vi "Write Lookup Tables.vi"(8 "error in (no error)":errorcluster, 10 "Lookup Tables":T1[](array[typedef]), 11 "Plugin_UI in":refnum<class "Plugin_UI.lvclass">) -> (0 "error out":errorcluster, 3 "Plugin_UI out":refnum<class "Plugin_UI.lvclass">)   [LabVIEW 2020, in "Plugin.lvlib" / "Plugin_UI.lvclass"]
doc: "Write lookup table"
uses:
  Plugin_UI.lvclass
  builds/Libraries/LabSys Framework.lvlibp/Configuration Storage/Test Configuration/Table Information.ctl
  Plugin_UI.lvclass/Plugin_UI.ctl
  builds/Libraries/LabSys Framework.lvlibp/Configuration Storage/Test Configuration/Test Configuration.lvclass
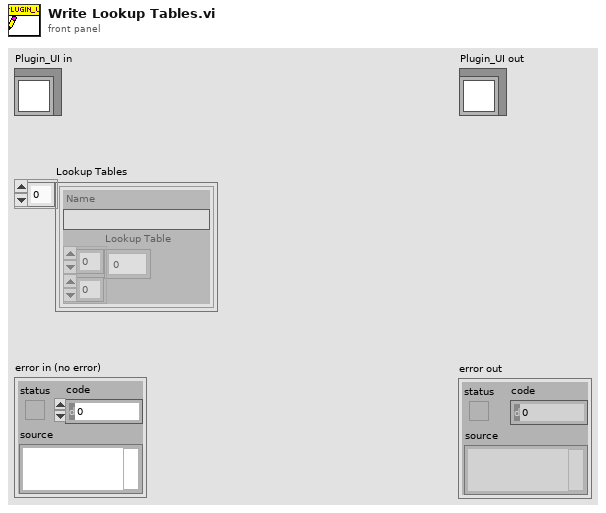
[diagram p1: front panel]
types:
  T1 = typedef "LabSys Framework.lvlibp/Configuration Storage.lvlib/Test Configuration.lvclass/Table Information.ctl" = cluster{"Name":string, "Lookup Table":dbl[][]}
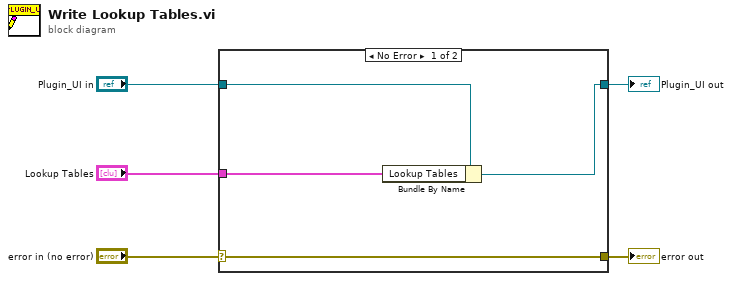
[diagram p0: block diagram]
diagram:
  n1 = case shown="No Error" "error in (no error)" {
    selector: "error in (no error)" -> [w9 w10]
    tunnel: [w9 w10] -> w4
    tunnel: [w7 w11] -> w2
    tunnel: "Plugin_UI in" -> [w8 w11]
    tunnel: "Lookup Tables" -> [w6 _]
    frame No Error {
      n2 = Bundle By Name(cluster=w8, "Lookup Tables"=w6) -> (w7:refnum<class "Plugin_UI.lvclass">)
    }
    frame Error {
    }
  }
  "error out" <- w4
  "Plugin_UI out" <- w2
